vi "test Clear Data.vi"(8 "error in (no error)":errorcluster, 11 "TestCase in":refnum<class "Data Manipulation Tests.lvclass">) -> (0 "error out":errorcluster, 3 "TestCase out":refnum<class "Data Manipulation Tests.lvclass">)   [LabVIEW 2027, in "Memory Manager Tests.lvlib" / "Data Manipulation Tests.lvclass"]
uses:
  Data Manipulation Tests.lvclass
  Classes/Pointer/Write 1D U8.vi
  Classes/Pointer/Read 1D U8.vi
  C:/Program Files/National Instruments/LabVIEW 2027/vi.lib/addons/_JKI Toolkits/VI Tester/TestCase.llb/TestCase.lvclass
  <vilib>/addons/_JKI Toolkits/VI Tester/TestCase.llb/TestCase.lvclass
  Classes/Pointer/Pointer.lvclass
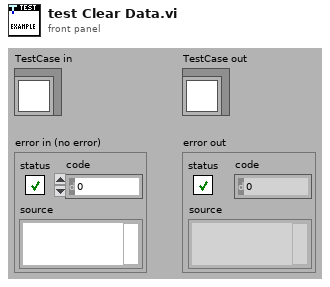
[diagram p1: front panel]
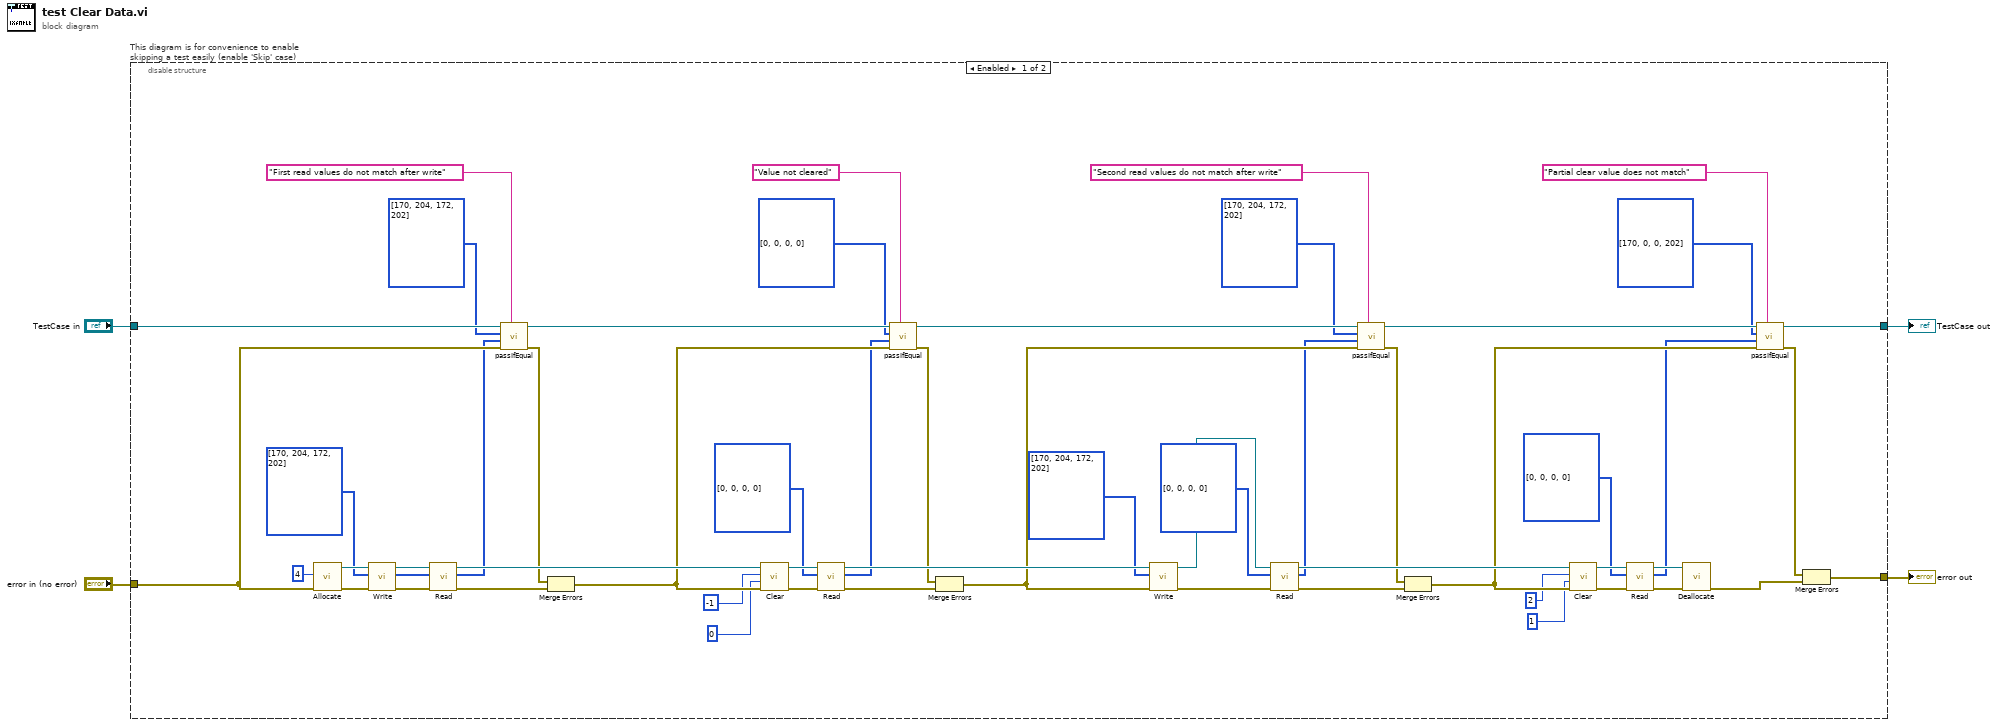
[diagram p0: block diagram]
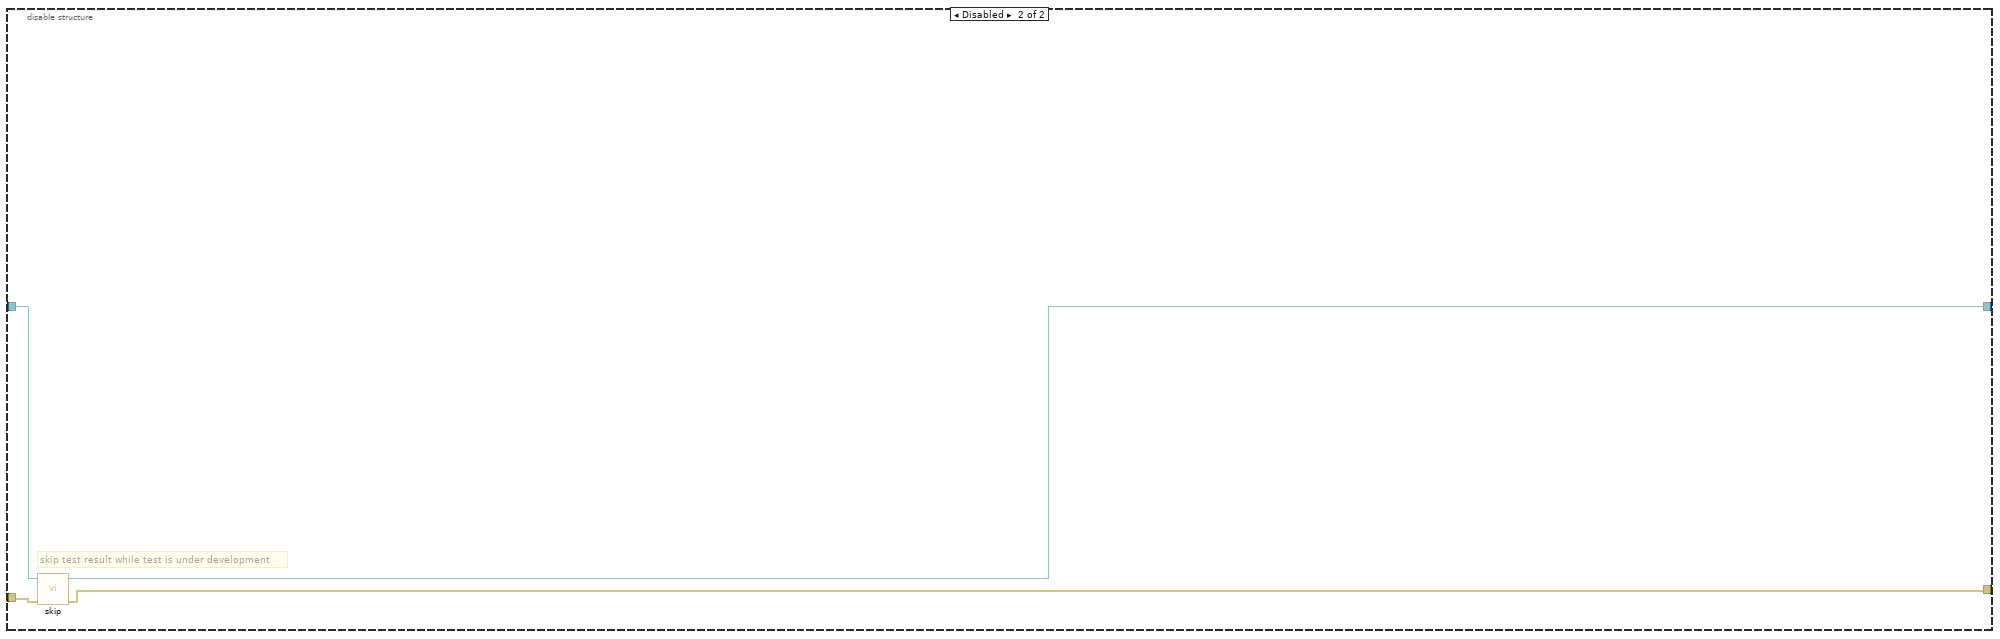
[diagram p2: hidden frame]
diagram:
  n1 = disable-structure "This diagram is for convenience to enable skipping a test easily (enable 'Skip' case)" shown="Enabled" {
    disable-tunnel: "TestCase in" -> [w56 w64]
    disable-tunnel: [w59 w62] -> w1
    disable-tunnel: [w58 w63] -> w3
    disable-tunnel: "error in (no error)" -> [w51 w61]
    frame Enabled {
      n2 = call "Allocate.vi"("error in (no error)"=w51, "size"=u64 4 ("count (1)")) -> ("error out"=w45:errorcluster, "Pointer out"=w47:refnum<class "Pointer.lvclass">)  [unwired: 8 in]
      n3 = call-poly "Write.vi"("error in (no error)"=w45, "buffer in"=u8[] [170, 204, 172, 202], "Pointer in"=w47) -> ("error out"=w44:errorcluster, "buffer out"=w13:u8[], "Pointer out"=w42:refnum<class "Pointer.lvclass">)  [unwired: 5 in, 1 out]
      n4 = call-poly "Read.vi"("error in (no error)"=w44, "buffer in"=w13, "Pointer in"=w42) -> ("error out"=w43:errorcluster, "buffer out"=w12:u8[], "Pointer out"=w57:refnum<class "Pointer.lvclass">)  [unwired: 5 in, 1 out]
      n5 = call-dynamic "passIfEqual.vi"("custom report message (\"\")"="First read values do not match after write" ("custom report message (\"\")"), "error in (no error)"=w51, "y"=w12, "x"=u8[] [170, 204, 172, 202] ("buffer in"), "TestCase in"=w56) -> ("error out"=w40:errorcluster, "TestCase out"=w55:refnum<class "Data Manipulation Tests.lvclass">)  [unwired: 5 in]
      n6 = Merge Errors(w40, w43) -> (w50:errorcluster)
      n7 = call "Clear.vi"("error in (no error)"=w50, "offset (0)"=u64 0, "length (-1: rest)"=i64 -1, "Pointer in"=w57) -> ("error out"=w38:errorcluster, "Pointer out"=w37:refnum<class "Pointer.lvclass">)  [unwired: 6 in]
      n8 = call-poly "Read.vi"("error in (no error)"=w38, "buffer in"=u8[] [0, 0, 0, 0], "Pointer in"=w37) -> ("error out"=w39:errorcluster, "buffer out"=w11:u8[], "Pointer out"=w60:refnum<class "Pointer.lvclass">)  [unwired: 5 in, 1 out]
      n9 = call-dynamic "passIfEqual.vi"("custom report message (\"\")"="Value not cleared" ("custom report message (\"\")"), "error in (no error)"=w50, "y"=w11, "x"=u8[] [0, 0, 0, 0] ("buffer in"), "TestCase in"=w55) -> ("error out"=w33:errorcluster, "TestCase out"=w53:refnum<class "Data Manipulation Tests.lvclass">)  [unwired: 5 in]
      n10 = Merge Errors(w33, w39) -> (w49:errorcluster)
      n11 = call-poly "Write.vi"("error in (no error)"=w49, "buffer in"=u8[] [170, 204, 172, 202], "Pointer in"=w60) -> ("error out"=w31:errorcluster, "Pointer out"=w29:refnum<class "Pointer.lvclass">)  [unwired: 5 in, 2 out]
      n12 = call-poly "Read.vi"("error in (no error)"=w31, "buffer in"=u8[] [0, 0, 0, 0], "Pointer in"=w29) -> ("error out"=w30:errorcluster, "buffer out"=w7:u8[], "Pointer out"=w54:refnum<class "Pointer.lvclass">)  [unwired: 5 in, 1 out]
      n13 = call-dynamic "passIfEqual.vi"("custom report message (\"\")"="Second read values do not match after write" ("custom report message (\"\")"), "error in (no error)"=w49, "y"=w7, "x"=u8[] [170, 204, 172, 202] ("buffer in"), "TestCase in"=w53) -> ("error out"=w27:errorcluster, "TestCase out"=w52:refnum<class "Data Manipulation Tests.lvclass">)  [unwired: 5 in]
      n14 = Merge Errors(w27, w30) -> (w48:errorcluster)
      n15 = call "Clear.vi"("error in (no error)"=w48, "offset (0)"=u64 1, "length (-1: rest)"=i64 2, "Pointer in"=w54) -> ("error out"=w23:errorcluster, "Pointer out"=w22:refnum<class "Pointer.lvclass">)  [unwired: 6 in]
      n16 = call-poly "Read.vi"("error in (no error)"=w23, "buffer in"=u8[] [0, 0, 0, 0], "Pointer in"=w22) -> ("error out"=w24:errorcluster, "buffer out"=w5:u8[], "Pointer out"=w17:refnum<class "Pointer.lvclass">)  [unwired: 5 in, 1 out]
      n17 = call "Deallocate.vi"("error in (no error)"=w24, "Pointer"=w17) -> ("error out"=w18:errorcluster)  [unwired: 8 in, 1 out]
      n18 = call-dynamic "passIfEqual.vi"("custom report message (\"\")"="Partial clear value does not match" ("custom report message (\"\")"), "error in (no error)"=w48, "y"=w5, "x"=u8[] [170, 0, 0, 202] ("buffer in"), "TestCase in"=w52) -> ("error out"=w25:errorcluster, "TestCase out"=w59:refnum<class "Data Manipulation Tests.lvclass">)  [unwired: 5 in]
      n19 = Merge Errors(w25, w18) -> (w58:errorcluster)
    }
    frame Disabled {
      # "skip test result while test is under development"
      n20 = call <vilib>:"skip.vi"("error in (no error)"=w61, "TestCase in"=w64) -> ("error out"=w63:errorcluster, "TestCase out"=w62:refnum<class "Data Manipulation Tests.lvclass">)  [unwired: 8 in]
    }
  }
  "error out" <- w3
  "TestCase out" <- w1
